vi "SCB.vi"(0 "States":refnum<vi>, 1 "VPInputMsgs":refnum<vi>, 2 "VMInputMsgs":refnum<vi>, 3 "SCM2VM":refnum<vi>, 4 "SCM2VP":refnum<vi>, 5 "ÑAInputMsgs":refnum<vi>, 6 "SCM2CA":refnum<vi>, 7 "Processes":refnum<vi>, 8 "SCBStates":refnum<vi>) -> ()   [LabVIEW 2010]
uses:
  lib/Ports.lvclass
panel:
  out "Output messages to VM":T1(array[cluster])
  out "Output messages to VP":T1(array[cluster])
  out "Output messages to CA":T1(array[cluster])
  out "States of processes:":string[][](table)
  # "Script control module"
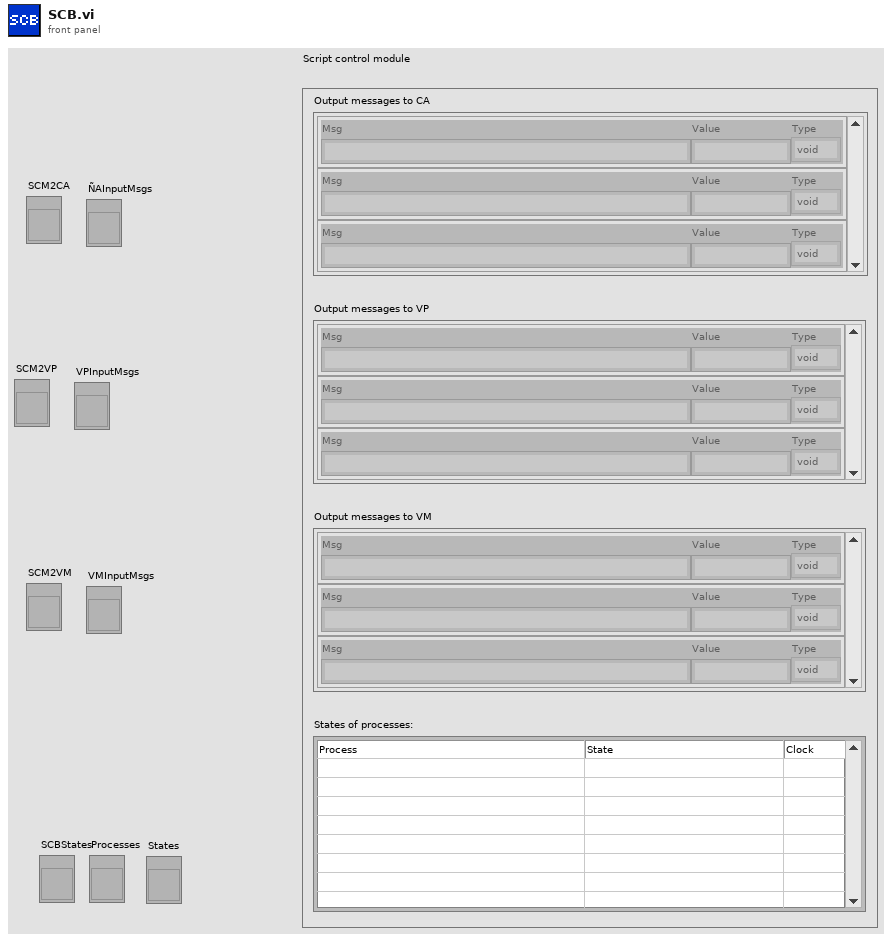
[diagram p1: front panel]
types:
  T1 = cluster{"Msg":string, "Value":string, "Type":enum16{"void", "byte", "int", "float"}}[]
  T2 = cluster{"Сообщение":string, "Значение":string, "Тип":enum16{"void", "byte", "int", "float"}}
  T3 = cluster{"Сообщение":string, "Значение":string, "Тип":enum16{"void", "byte", "int", "float"}}[]
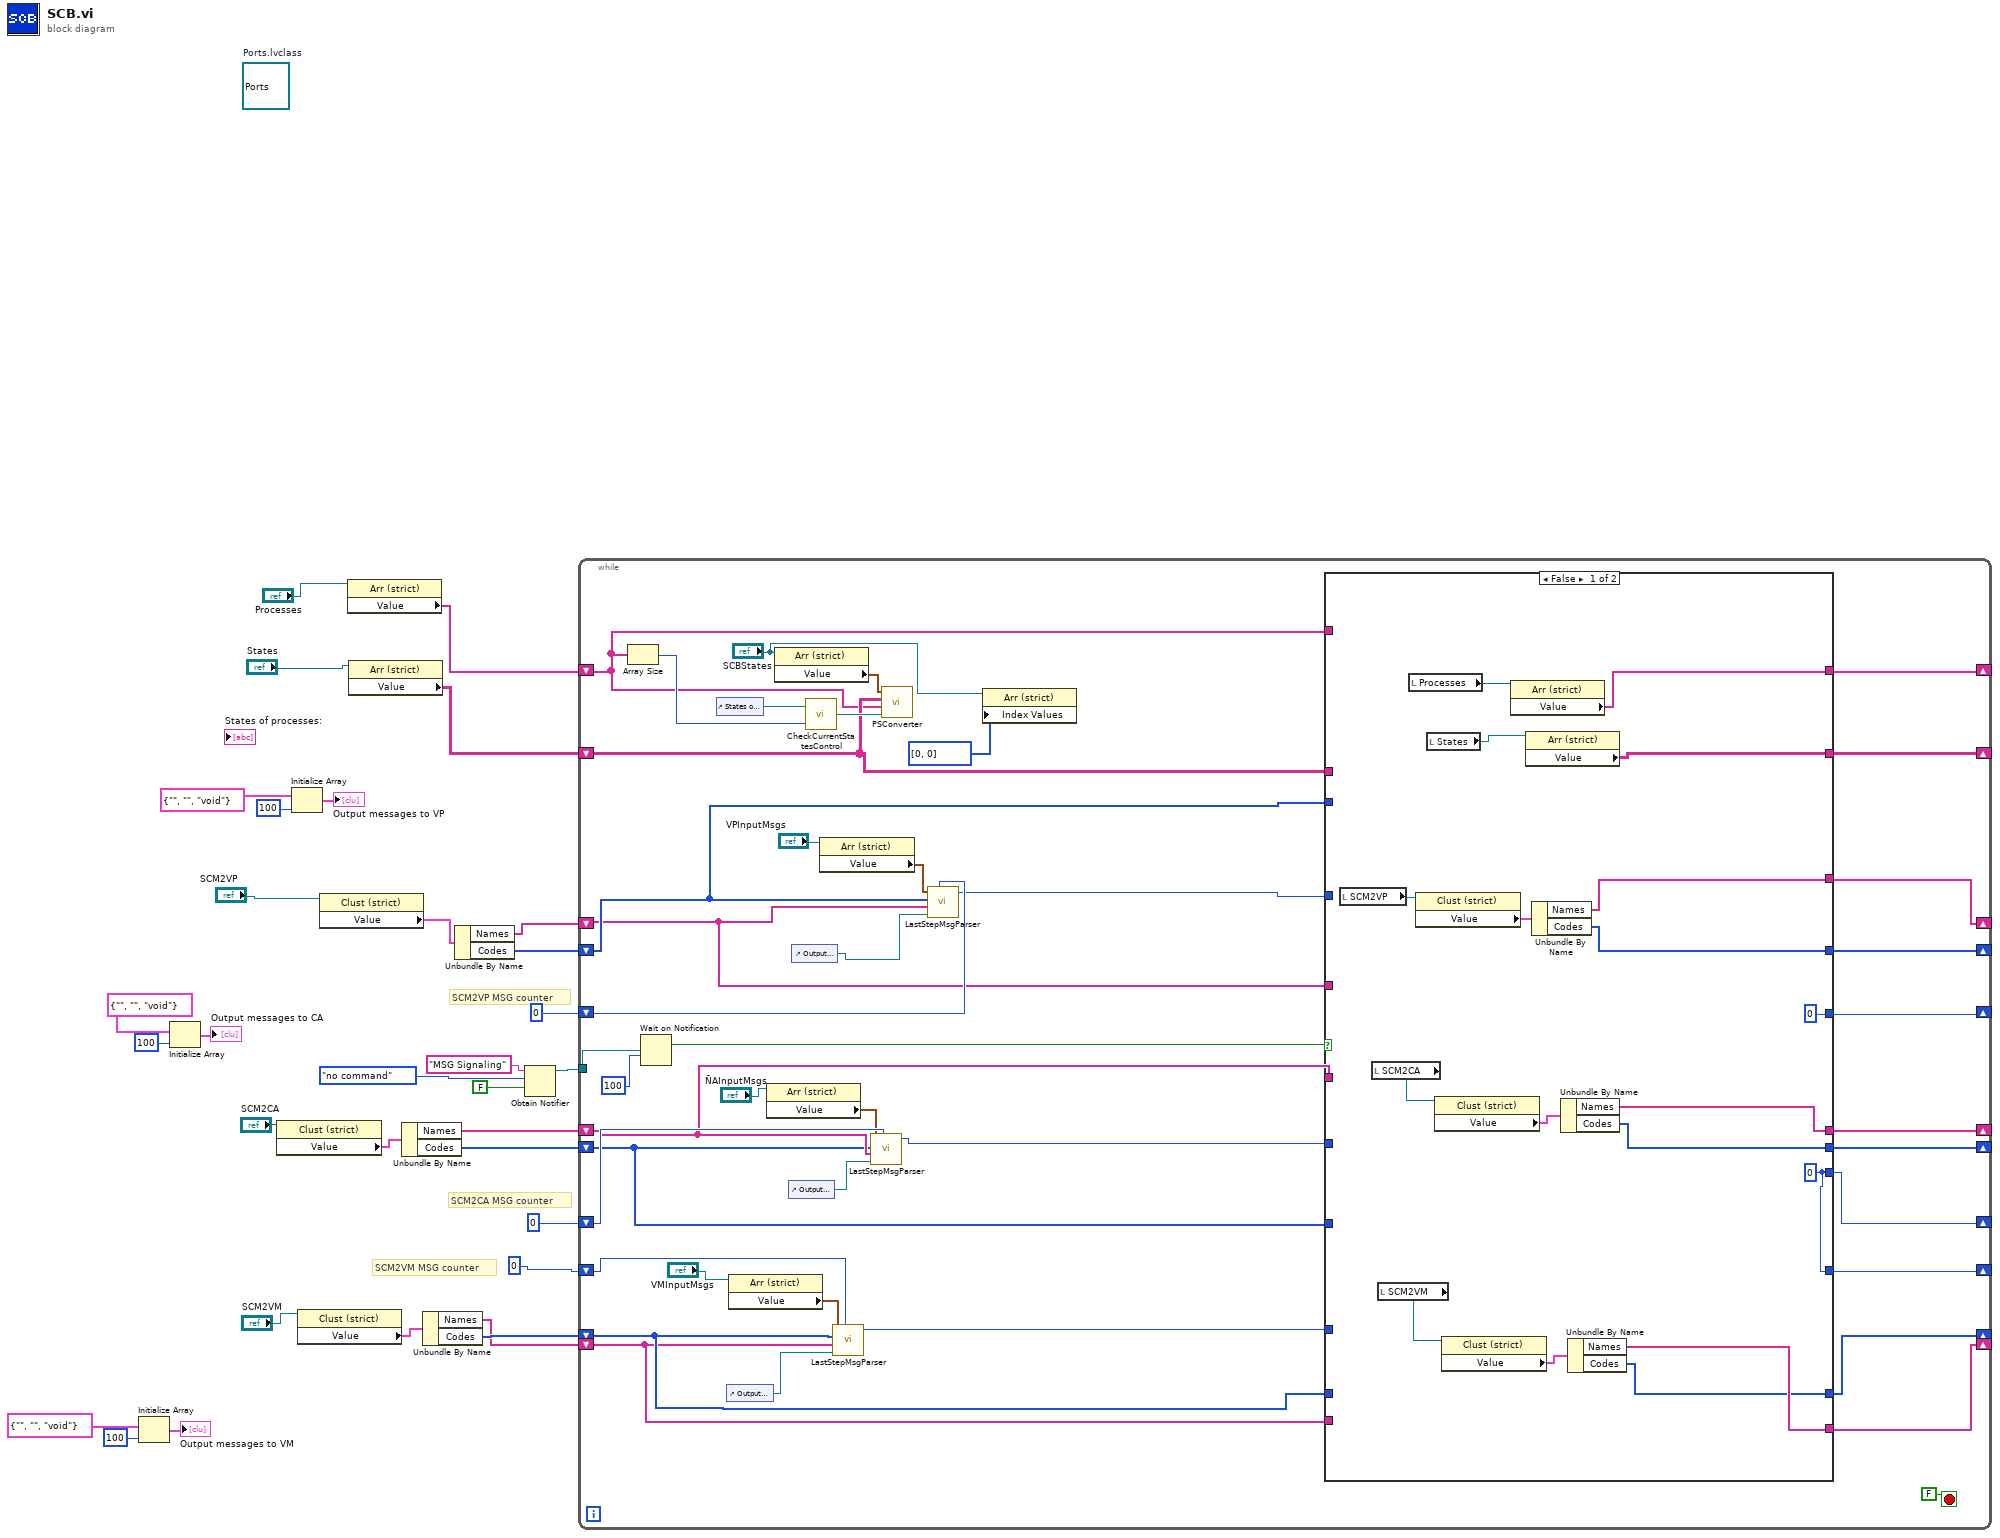
[diagram p0: block diagram]
diagram:
  (unwired) refnum<class "Ports.lvclass"> refnum  # Ports.lvclass
  # "SCM2VM MSG counter"
  # "SCM2CA MSG counter"
  # "SCM2VP MSG counter"
  n1 = Initialize Array(T2 {"Сообщение"="", "Значение"="", "Тип"=enum."void"} ("Cluster"), 100 ("dimension size")) -> (→"Output messages to VM":T3)
  n2 = Initialize Array(T2 {"Сообщение"="", "Значение"="", "Тип"=enum."void"} ("Cluster"), 100 ("dimension size")) -> (→"Output messages to CA":T3)
  n3 = property class="Clust (strict)"(reference="SCM2CA") -> ("Value"=w9:cluster{"Names":string[], "Codes":i32[]})  [unwired: 1 in, 2 out]
  n4 = Initialize Array(T2 {"Сообщение"="", "Значение"="", "Тип"=enum."void"} ("Cluster"), 100 ("dimension size")) -> (→"Output messages to VP":T3)
  n5 = property class="Clust (strict)"(reference="SCM2VM") -> ("Value"=w5:cluster{"Names":string[], "Codes":i32[]})  [unwired: 1 in, 2 out]
  n6 = property class="Clust (strict)"(reference="SCM2VP") -> ("Value"=w27:cluster{"Names":string[], "Codes":i32[]})  [unwired: 1 in, 2 out]
  n7 = property class="Arr (strict)"(reference="Processes") -> ("Value"=w30:string[])  [unwired: 1 in, 2 out]
  n8 = property class="Arr (strict)"(reference="States") -> ("Value"=w29:string[][])  [unwired: 1 in, 2 out]
  n9 = Unbundle By Name(w9) -> ("Names"=w8:string[], "Codes"=w7:i32[])
  n10 = Unbundle By Name(w5) -> ("Names"=w1:string[], "Codes"=w2:i32[])
  n11 = Unbundle By Name(w27) -> ("Names"=w26:string[], "Codes"=w25:i32[])
  n12 = Obtain Notifier(name (unnamed)="MSG Signaling", notification data type=enum16{"no command", "refresh"}."no command", create if not found? (T)=FALSE) -> (notifier out=w17:refnum<notifier>)  [unwired: 1 in, 2 out]
  n13 = while {
    shift-right: [w65] -> _
    shift-left: 0 ("dimension size") -> [w68]
    tunnel: w17 -> [w67]
    shift-right: [w63] -> _
    shift-left: w25 -> [w64]
    shift-right: [w62] -> _
    shift-left: w26 -> [w61]
    shift-right: [w56] -> _
    shift-left: w29 -> [w59]
    shift-right: [w57] -> _
    shift-left: w30 -> [w58]
    shift-right: [w47] -> _
    shift-left: w8 -> [w45]
    shift-right: [w46] -> _
    shift-left: w7 -> [w44]
    shift-right: [w51] -> _
    shift-left: 0 ("dimension size") -> [w53]
    shift-right: [w38] -> _
    shift-left: 0 ("dimension size") -> [w41]
    shift-right: [w37] -> _
    shift-left: w2 -> [w36]
    shift-right: [w34] -> _
    shift-left: w1 -> [w35]
    stop <- FALSE ("stop") stop-if-true
    n14 = Array Size(array=w58) -> (size(s)=w60:i32)
    n15 = Wait on Notification(notifier=w67, timeout in ms (-1)=100) -> (timed out?=w48:bool)  [unwired: 2 in, 3 out]
    n16 = control-ref of="States of processes:"() -> (w75:refnum<vi>)
    n17 = control-ref of="Output messages to VM"() -> (w40:refnum<vi>)
    n18 = property class="Arr (strict)"(reference="VMInputMsgs") -> ("Value"=w43:cluster{"MSG":i16, "param":i32, "Type":i16}[])  [unwired: 1 in, 2 out]
    n19 = property class="Arr (strict)"(reference="ÑAInputMsgs") -> ("Value"=w49:cluster{"MSG":i16, "param":i32, "Type":i16}[])  [unwired: 1 in, 2 out]
    n20 = property class="Arr (strict)"(reference="SCBStates") -> ("Value"=w76:cluster{"TimeInState":u16, "cur_state":i8}[])  [unwired: 1 in, 2 out]
    n21 = control-ref of="Output messages to CA"() -> (w54:refnum<vi>)
    n22 = control-ref of="Output messages to VP"() -> (w33:refnum<vi>)
    n23 = call "CheckCurrentStatesControl.vi"("Processes"=w60, "Inp reference"=w75) -> ("Out Refnum"=w74:refnum<vi>)
    n24 = property class="Arr (strict)"(reference="VPInputMsgs") -> ("Value"=w69:cluster{"MSG":i16, "param":i32, "Type":i16}[])  [unwired: 1 in, 2 out]
    n25 = call "LastStepMsgParser.vi"("Arr Refnum"=w40, "Out MSG Names"=w35, "old msg counter"=w41, "Codes"=w36, "Msg Array"=w43) -> ("current msg counter"=w39:i32)  [unwired: 4 in, 1 out]
    n26 = call "LastStepMsgParser.vi"("Arr Refnum"=w54, "Out MSG Names"=w45, "old msg counter"=w53, "Codes"=w44, "Msg Array"=w49) -> ("current msg counter"=w52:i32)  [unwired: 4 in, 1 out]
    n27 = call "PSConverter.vi"("Tbl Refnum"=w74, "PROC"=w58, "STATES"=w59, "Input claster"=w76) -> ()  [unwired: 1 out]
    n28 = call "LastStepMsgParser.vi"("Arr Refnum"=w33, "Out MSG Names"=w61, "old msg counter"=w68, "Codes"=w64, "Msg Array"=w69) -> ("current msg counter"=w66:i32)  [unwired: 4 in, 1 out]
    n29 = property class="Arr (strict)"(reference="SCBStates", "Index Values"=u32[] [0, 0]) -> ()  [unwired: 1 in, 2 out]
    n30 = case shown="False" w48 {
      tunnel: w66 -> [_ w103]
      tunnel: [0 ("current msg counter") w103] -> w65
      tunnel: w64 -> [_ w105]
      tunnel: [w90 w105] -> w63
      tunnel: [w91 w104] -> w62
      tunnel: w61 -> [_ w104]
      tunnel: w59 -> [_ w101]
      tunnel: w58 -> [_ w102]
      tunnel: [w88 w102] -> w57
      tunnel: [w86 w101] -> w56
      tunnel: w52 -> [_ w100]
      tunnel: [w78 w100] -> w51
      tunnel: [w83 w99] -> w47
      tunnel: [w82 w98] -> w46
      tunnel: w45 -> [_ w99]
      tunnel: w44 -> [_ w98]
      tunnel: w39 -> [_ w97]
      tunnel: [w78 w97] -> w38
      tunnel: [w79 w96] -> w37
      tunnel: w36 -> [_ w96]
      tunnel: w35 -> [_ w95]
      tunnel: [w80 w95] -> w34
      frame False {
        w78 = 0 ("current msg counter")
        n31 = local read "SCM2VP"() -> (w93:refnum<vi>)
        n32 = local read "SCM2CA"() -> (w84:refnum<vi>)
        n33 = local read "SCM2VM"() -> (w77:refnum<vi>)
        n34 = local read "Processes"() -> (w89:refnum<vi>)
        n35 = property class="Clust (strict)"(reference=w93) -> ("Value"=w92:cluster{"Names":string[], "Codes":i32[]})  [unwired: 1 in, 2 out]
        n36 = local read "States"() -> (w87:refnum<vi>)
        n37 = property class="Clust (strict)"(reference=w84) -> ("Value"=w85:cluster{"Names":string[], "Codes":i32[]})  [unwired: 1 in, 2 out]
        n38 = property class="Clust (strict)"(reference=w77) -> ("Value"=w81:cluster{"Names":string[], "Codes":i32[]})  [unwired: 1 in, 2 out]
        n39 = property class="Arr (strict)"(reference=w89) -> ("Value"=w88:string[])  [unwired: 1 in, 2 out]
        n40 = property class="Arr (strict)"(reference=w87) -> ("Value"=w86:string[][])  [unwired: 1 in, 2 out]
        n41 = Unbundle By Name(w92) -> ("Names"=w91:string[], "Codes"=w90:i32[])
        n42 = Unbundle By Name(w85) -> ("Names"=w83:string[], "Codes"=w82:i32[])
        n43 = Unbundle By Name(w81) -> ("Names"=w80:string[], "Codes"=w79:i32[])
      }
      frame True {
      }
    }
  }
